vi "Send Message Without Read.vi"(6 "Timeout (25000)":u32=25000, 8 "error in (no error)":errorcluster, 10 "Send Message (\"\")":string, 11 "VISA resource name":refnum<visa-resource-name>) -> (0 "error out":errorcluster, 3 "VISA resource name out":refnum<visa-resource-name>)   [LabVIEW 2020, in "Yokogawa GX Series.lvlib"]
doc: "This VI sends the message. Then it returns the response."
uses:
  <instrlib>/Yokogawa GX Series/Yokogawa GX Series.lvlib
panel:
  # "msec"
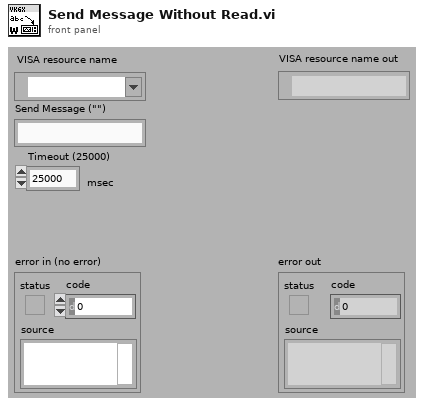
[diagram p1: front panel]
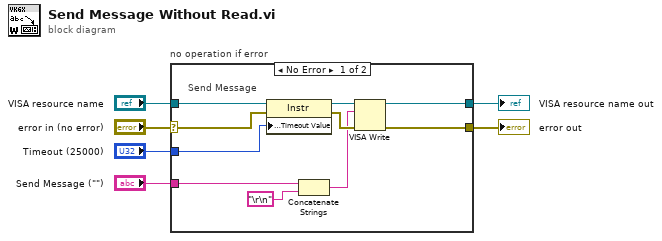
[diagram p0: block diagram]
diagram:
  n1 = case "no operation if error" shown="No Error" "error in (no error)" {
    selector: "error in (no error)" -> [w12 w17]
    tunnel: "VISA resource name" -> [w15 w18]
    tunnel: "Send Message (\"\")" -> [w9 _]
    tunnel: [w8 w18] -> w4
    tunnel: [w7 w17] -> w6
    tunnel: "Timeout (25000)" -> [w13 _]
    frame No Error {
      # "Send Message"
      n2 = property class="Instr"(reference=w15, error in=w12, "General Settings:Timeout Value"=w13) -> (reference out=w14:refnum<visa-resource-name>, error out=w16:errorcluster)
      n3 = Concatenate Strings(w9, "\r\n") -> (w10:string)
      n4 = VISA Write(VISA resource name=w14, write buffer=w10, error in (no error)=w16) -> (VISA resource name out=w8:refnum<visa-resource-name>, error out=w7:errorcluster)  [unwired: 1 out]
    }
    frame Error {
    }
  }
  "error out" <- w6
  "VISA resource name out" <- w4
